vi "API_DB.FindFirstSlot.vi"(6 "Timeout (ms)":u32, 7 "Wait (F)":bool, 8 "error in (no error)":errorcluster, 11 "Database in":refnum<class "Database.lvclass">) -> (0 "error out":errorcluster, 2 "Slot":string, 3 "Database out":refnum<class "Database.lvclass">)   [LabVIEW 2022 SP3, in "Database.lvclass"]
doc: "Developed by Kevin Thompson\nkevin@thompsonengineering.net\n\nCopyright 2018\nThompson Engineering, LLC"
uses:
  Database.lvclass
  DataTypes/AsynCmd_Temp01--enum.ctl
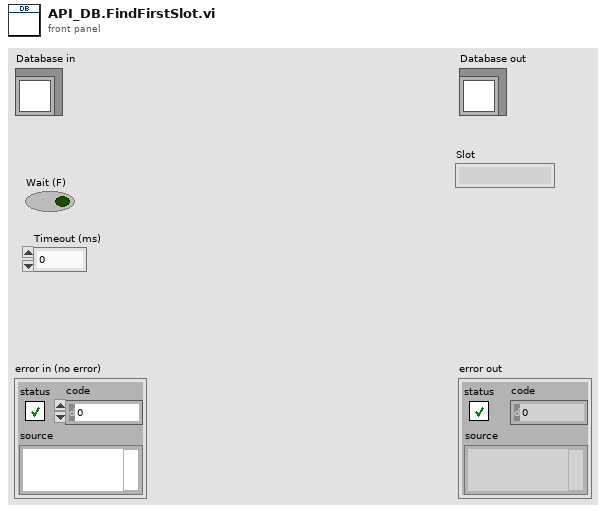
[diagram p1: front panel]
types:
  T1 = typedef "Database.lvclass/AsynCmd_Temp01--enum.ctl" = enum16{"DB.DeleteRecord", "DB.UpdateRecord", "DB.InsertRecord", "DB.SelectRecord", "DB.ExecuteSQLCommand", "DB.FindFirstSlot", "DB.GenericSQLQuery"}
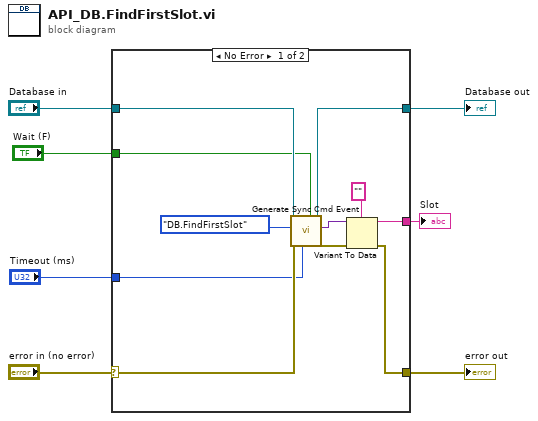
[diagram p0: block diagram]
diagram:
  n1 = case shown="No Error" "error in (no error)" {
    selector: "error in (no error)" -> [w16 w20]
    tunnel: [w11 w20] -> w6
    tunnel: [w17 w19] -> w4
    tunnel: "Database in" -> [w18 w19]
    tunnel: [w13 _] -> w1
    tunnel: "Wait (F)" -> [w10 _]
    tunnel: "Timeout (ms)" -> [w9 _]
    frame No Error {
      n2 = call "Generate Sync Cmd Event.vi"("Wait (F)"=w10, "Timeout (ms)"=w9, "error in (no error)"=w16, "AsyncCmd"=AsynCmd_Temp01--enum."DB.FindFirstSlot", "Database in"=w18) -> ("error out"=w12:errorcluster, "Return Value"=w14:variant, "Database out"=w17:refnum<class "Database.lvclass">)  [unwired: 4 in]
      n3 = Variant To Data(error in=w12, type="", Variant=w14) -> (data=w13:string, error out=w11:errorcluster)
    }
    frame Error {
    }
  }
  "error out" <- w6
  "Database out" <- w4
  "Slot" <- w1
